vi "读取.vi"() -> ()   [LabVIEW 2018]
panel:
  out "波形图":i32[][](graph)
  out "表格控件":string[][](table)
  out "数组":i32[][](array[numeric])
  out "文本":string
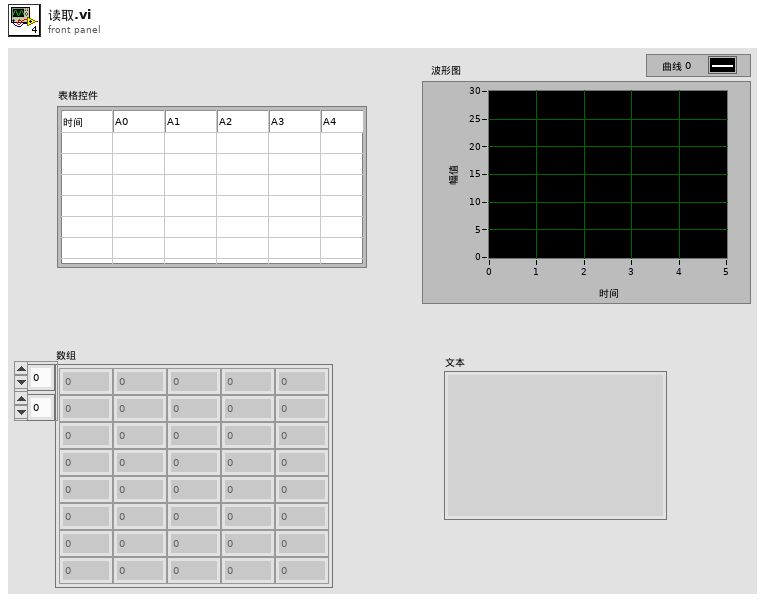
[diagram p1: front panel]
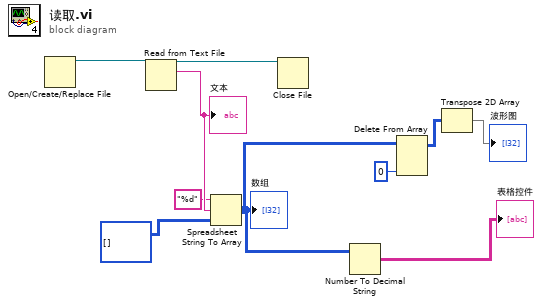
[diagram p0: block diagram]
diagram:
  n1 = Open/Create/Replace File() -> (refnum out=w10:refnum<file>)  [unwired: 6 in, 2 out]
  n2 = Read from Text File(file (use dialog)=w10) -> (refnum out=w9:refnum<file>, text=w8:string)  [unwired: 3 in, 2 out]
  "文本" <- w8
  n3 = Spreadsheet String To Array(format string="%d" ("格式字符串"), spreadsheet string=w8, array type (2D Dbl)=i32[][] []) -> (array=w4:i32[][])  [unwired: 1 in]
  "数组" <- w4
  n4 = Close File(refnum=w9) -> ()  [unwired: 1 in, 2 out]
  n5 = Number To Decimal String(number=w4) -> (decimal integer string=→"表格控件":string[][])  [unwired: 1 in]
  n6 = Delete From Array(array=w4, index (col)=0 ("禁用的索引 (列)")) -> (array with subset deleted=w2:i32[][])  [unwired: 2 in, 1 out]
  n7 = Transpose 2D Array(2D array=w2) -> (transposed array=→"波形图":i32[][])
